vi "XNET BM Iterate Frame Raw to CAN.vi"(5 "index in":i32, 7 "raw frames":u8[](array[numeric]) format="%02x", 11 "error in":errorcluster) -> (4 "output BM Frame":T1={"timestamp"=timestamp(0 s since 1904-01-01), "payload"=[0, 0, 0, 0, 0, 0, 0, 0], "identifier / slot"=0, "Data type"=0, "payload length"=0, "CAN"={"extended?"=FALSE}, "FlexRay"={"cycle count"=0, "startup?"=FALSE, "sync?"=FALSE, "preamble?"=FALSE, "ch A"=FALSE, "ch B"=FALSE, "macrotick"=32}, "echo?"=FALSE} {"FlexRay"."cycle count" max=63 step=1; "payload" format="%x"; "identifier / slot" format="%x"}, 6 "index out":i32, 10 "valid?":bool, 15 "error out":errorcluster)   [LabVIEW 2014, in "CAN Bus Monitor Engine.lvlib"]
doc: "Iterate array of raw frame data to extract a single CAN frame.\n\nIndex in specifies the start of the new CAN frame in the raw data. If no valid frame exists at this index, the boolean \"valid?\" is false.\n\nIndex out specfies the start of the next CAN frame in raw data, or -1 if the end of the raw data was reached.\n\nThis VI is part of the NI-XNET example set."
uses:
  CAN Bus Monitor Engine.lvlib
  Controls/XNET BM Frame.ctl
  <vilib>/xnet/xnet.llb/XNET Frame Type CAN.ctl
  Controls/Set Dyn Vars.ctl
  BM Global Vars.vi
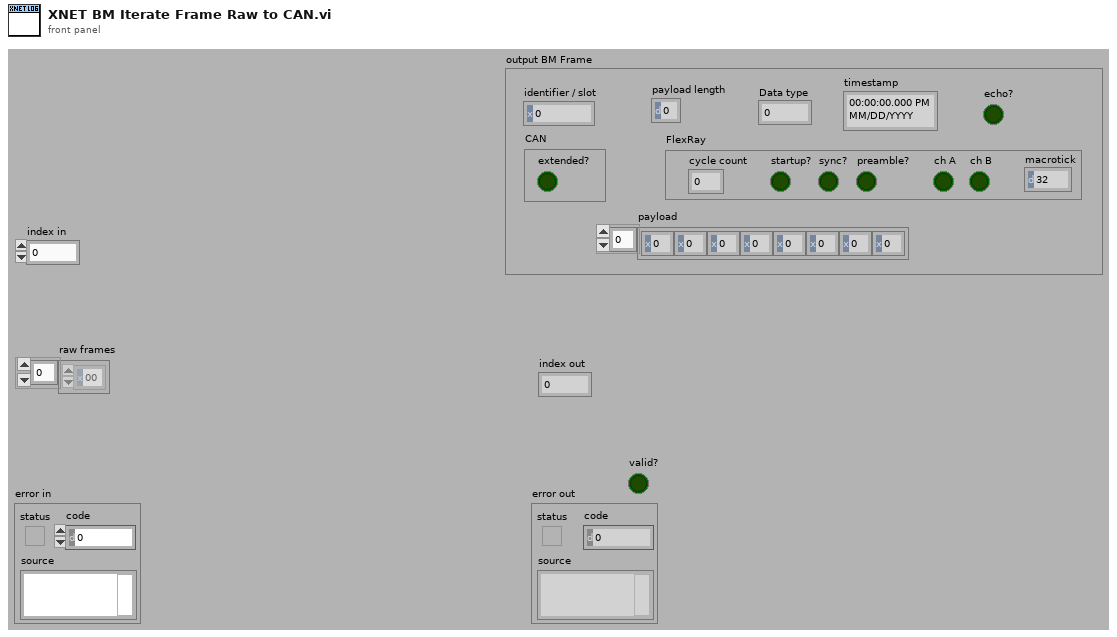
[diagram p1: front panel]
types:
  T1 = typedef "CAN Bus Monitor Engine.lvlib/XNET BM Frame.ctl" = cluster{"timestamp":timestamp, "payload":u8[], "identifier / slot":u32, "Data type":u8, "payload length":u8, "CAN":cluster{"extended?":bool}, "FlexRay":cluster{"cycle count":u8, "startup?":bool, "sync?":bool, "preamble?":bool, "ch A":bool, "ch B":bool, "macrotick":u16}, "echo?":bool}
  T2 = typedef "CAN Bus Monitor Engine.lvlib/Set Dyn Vars.ctl" = enum16{"Std Frames", "Std Frames / Sec", "Ext Frames", "Ext Frames / Sec", "Remote Frames", "Remote Frames / Sec", "Error Frames", "Error Frames / Sec", "BusLoad", "SumFrames", "SumFrames / Sec", "Null Frames", "Null Frames / Sec", "Peak Bus Load", "State", "IncMinFrameTime", "IncMaxFrameTime", "Driver Status", "CAN Comm State", "LIN Comm State", "FlexRay Comm State"}
  T3 = typedef "XNET Frame Type CAN.ctl" = u8
  T4 = enum16{"big-endian, network order", "native, host order", "little-endian"}
  T5 = cluster{"IncMinFrameTime":dbl, "IncMaxFrameTime":dbl, "Min Frame Length":dbl[][], "Max Frame Length":dbl[][], "Std Frames":u32, "Ext Frames":u32, "Error Frames":u32, "Remote Frames":u32, "Std Frames / Sec":u32, "Ext Frames / Sec":u32, "Error Frames / Sec":u32, "Remote Frames / Sec":u32, "Peak Bus Load":dbl, "Bus Load":dbl, "Start Timestamp":dbl, "Null Frames":u32, "Null Frames / Sec":u32}
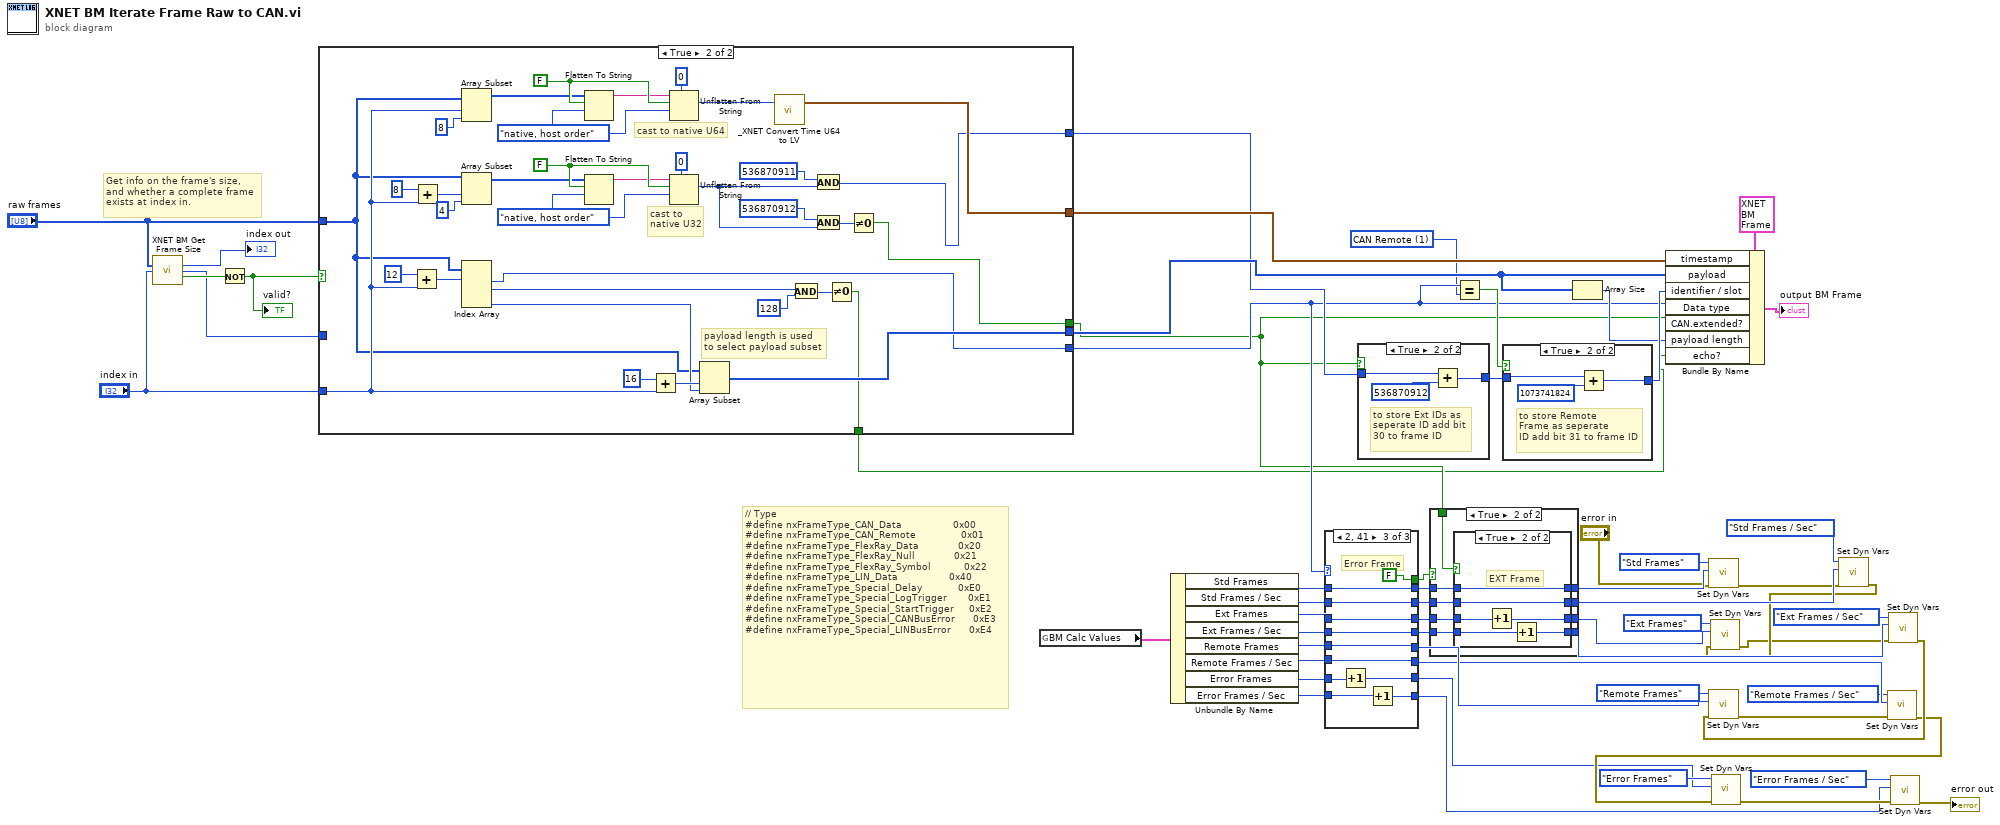
[diagram p0: block diagram]
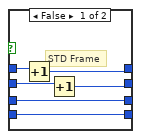
[diagram p3: hidden frame]
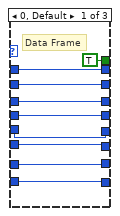
[diagram p6: hidden frame]
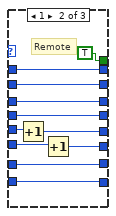
[diagram p7: hidden frame]
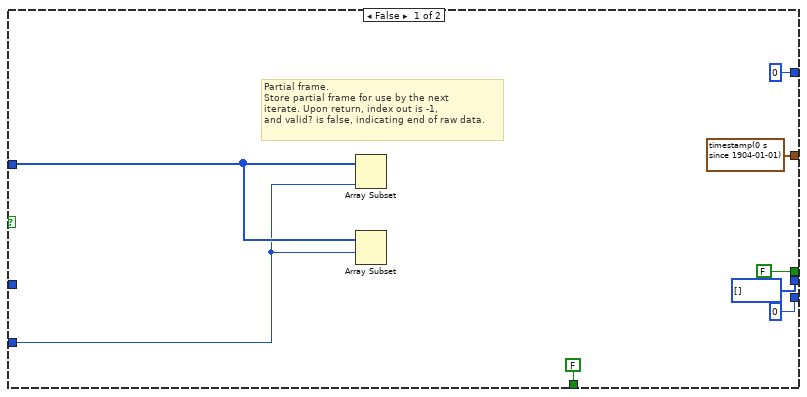
[diagram p8: hidden frame]
diagram:
  w31 = T3 1 items=["CAN Data", "CAN Remote"] ("type")
  # "// Type\n#define nxFrameType_CAN_Data                 0x00\n#define nxFrameType_CAN_Remote               0x01\n#define nxFrameType_FlexRay_Data             0x20\n#define nxFrameType_FlexRay_Null             0x21\n#define nxFrameType_FlexRay_Symbol           0x22\n#define nxFrameType_LIN_Data                 0x40\n#define nxFrameType_Special_Delay            0xE0\n#define nxFrameType_Special_LogTrigger       0xE1\n#define nxFrameType_Special_StartTrigger     0xE2\n#define nxFrameType_Special_CANBusError      0xE3\n#define nxFrameType_Special_LINBusError      0xE4"
  # "Get info on the frame's size,\nand whether a complete frame\nexists at index in."
  n1 = call "XNET BM Get Frame Size.vi"("raw frames"="raw frames", "index"="index in") -> ("next index"=→"index out":i32, "size"=w53:i32, "partial?"=w55:bool)  [unwired: 11 in]
  n2 = Not(x=w55) -> (.not. x?=w54:bool)
  "valid?" <- w54
  n3 = case shown="True" w54 {
    tunnel: "index in" -> [w65 w77]
    tunnel: "raw frames" -> [w66 w76]
    tunnel: w53 -> [_ _]
    tunnel: [timestamp(0 s since 1904-01-01) ("Time LV") w72] -> w37
    tunnel: [u8[] [] w71] -> w36
    tunnel: [u32 0 w70] -> w35
    tunnel: [u8 0 ("Numeric") w69] -> w34
    tunnel: [FALSE w68] -> w33
    tunnel: [FALSE w67] -> w1
    frame False {
      # "Partial frame.\nStore partial frame for use by the next \niterate. Upon return, index out is -1,\nand valid? is false, indicating end of raw data."
      n4 = Array Subset(array=w66, length=w65) -> ()  [unwired: 1 in, 1 out]
      n5 = Array Subset(array=w66, index=w65) -> ()  [unwired: 1 in, 1 out]
    }
    frame True {
      w82 = T4."native, host order" ("byte order (0:big-endian, network order)")
      w88 = T4."native, host order" ("byte order (0:big-endian, network order)")
      w83 = FALSE ("prepend array or string size? (T)")
      w89 = FALSE ("prepend array or string size? (T)")
      # "payload length is used\nto select payload subset"
      # "cast to \nnative U32"
      # "cast to native U64"
      n6 = Add(x=12, y=w77) -> (x+y=w93:i32)
      n7 = Add(x=8, y=w77) -> (x+y=w95:i32)
      n8 = Array Subset(array=w76, index=w77, length=8) -> (w80:u8[])
      n9 = Array Subset(array=w76, index=w95, length=4) -> (w86:u8[])
      n10 = Index Array(array=w76, index #1=w93) -> (element #1=w69:u8, element #2=w73:u8, element #4=w90:u8)  [unwired: 3 in, 1 out]
      n11 = Flatten To String(anything=w80, prepend array or string size? (T)=w83, byte order (0:big-endian, network order)=w82) -> (data string=w81:string)  [unwired: 1 in, 2 out]
      n12 = Flatten To String(anything=w86, prepend array or string size? (T)=w89, byte order (0:big-endian, network order)=w88) -> (data string=w87:string)  [unwired: 1 in, 2 out]
      n13 = Add(x=16, y=w77) -> (x+y=w91:i32)
      n14 = Unflatten From String(type=u64 0 ("length"), binary string=w81, data includes array or string size? (T)=w83, byte order (0:big-endian, network order)=w82) -> (value=w78:u64)  [unwired: 1 in, 2 out]
      n15 = Unflatten From String(type=u32 0 ("length"), binary string=w87, data includes array or string size? (T)=w89, byte order (0:big-endian, network order)=w88) -> (value=w84:u32)  [unwired: 1 in, 2 out]
      n16 = Array Subset(array=w76, index=w91, length=w90) -> (w71:u8[])
      n17 = call <vilib>:"_XNET Convert Time U64 to LV.vi"("Time U64"=w78) -> ("Time LV"=w72:timestamp)  [unwired: 2 in]
      n18 = And(x=w73, y=u8 128) -> (x .and. y?=w75:u8)
      n19 = And(x=u32 536870911, y=w84) -> (x .and. y?=w70:u32)
      n20 = And(x=u32 536870912, y=w84) -> (x .and. y?=w99:u32)
      n21 = Not Equal To 0?(x=w75) -> (x != 0?=w67:bool)
      n22 = Not Equal To 0?(x=w99) -> (x != 0?=w68:bool)
    }
  }
  n23 = global read "BM Global Vars.vi" "BM Calc Values"() -> (w30:T5)
  n24 = Unbundle By Name(w30) -> ("Std Frames"=w52:u32, "Std Frames / Sec"=w51:u32, "Ext Frames"=w50:u32, "Ext Frames / Sec"=w49:u32, "Remote Frames"=w48:u32, "Remote Frames / Sec"=w47:u32, "Error Frames"=w11:u32, "Error Frames / Sec"=w10:u32)
  n25 = case shown="2, 41" w34 {
    tunnel: w50 -> [w106 w119 w130]
    tunnel: w49 -> [w105 w118 w129]
    tunnel: w52 -> [w108 w121 w132]
    tunnel: [w108 w121 w132] -> w42
    tunnel: [w107 w120 w131] -> w41
    tunnel: w51 -> [w107 w120 w131]
    tunnel: [w106 w119 w130] -> w40
    tunnel: [w105 w118 w129] -> w39
    tunnel: w48 -> [w109 w117 w128]
    tunnel: w47 -> [w110 w116 w127]
    tunnel: [w109 w115 w128] -> w26
    tunnel: [w110 w114 w127] -> w25
    tunnel: w11 -> [w104 w113 w126]
    tunnel: w10 -> [w103 w112 w125]
    tunnel: [w104 w113 w124] -> w4
    tunnel: [w103 w112 w123] -> w3
    tunnel: [TRUE TRUE FALSE] -> w2
    frame 0, Default {
      # "Data Frame"
    }
    frame 1 {
      # "Remote"
      n26 = Increment(x=w117) -> (x+1=w115:u32)
      n27 = Increment(x=w116) -> (x+1=w114:u32)
    }
    frame 2, 65 {
      # "Error Frame"
      n28 = Increment(x=w126) -> (x+1=w124:u32)
      n29 = Increment(x=w125) -> (x+1=w123:u32)
    }
  }
  n30 = case shown="True" w33 {
    tunnel: w35 -> [w133 w135]
    tunnel: [w133 w136] -> w46
    frame False {
    }
    frame True {
      # "to store Ext IDs as\nseperate ID add bit \n30 to frame ID"
      n31 = Add(x=w135, y=u32 536870912) -> (x+y=w136:u32)
    }
  }
  n32 = case shown="True" w2 {
    tunnel: w42 -> [w140 w149]
    tunnel: w41 -> [w139 w148]
    tunnel: w40 -> [w138 w147]
    tunnel: w39 -> [w137 w146]
    tunnel: w33 -> [_ w145]
    tunnel: [w140 w144] -> w29
    tunnel: [w139 w143] -> w28
    tunnel: [w138 w142] -> w27
    tunnel: [w137 w141] -> w24
    frame False {
    }
    frame True {
      n33 = case shown="True" w145 {
        tunnel: w146 -> [w155 w161]
        tunnel: [w154 w160] -> w142
        tunnel: [w155 w159] -> w141
        tunnel: w147 -> [w154 w158]
        tunnel: w149 -> [w153 w157]
        tunnel: [w152 w157] -> w144
        tunnel: [w150 w156] -> w143
        tunnel: w148 -> [w151 w156]
        frame False {
          # "STD Frame"
          n34 = Increment(x=w153) -> (x+1=w152:u32)
          n35 = Increment(x=w151) -> (x+1=w150:u32)
        }
        frame True {
          # "EXT Frame"
          n36 = Increment(x=w158) -> (x+1=w160:u32)
          n37 = Increment(x=w161) -> (x+1=w159:u32)
        }
      }
    }
  }
  n38 = Equal?(x=w34, y=w31) -> (x = y?=w44:bool)
  n39 = case shown="True" w44 {
    tunnel: w46 -> [w162 w164]
    tunnel: [w162 w165] -> w45
    frame False {
    }
    frame True {
      # "to store Remote \nFrame as seperate \nID add bit 31 to frame ID"
      n40 = Add(x=w164, y=u32 1073741824) -> (x+y=w165:u32)
    }
  }
  n41 = Array Size(array=w36) -> (size(s)=w43:i32)
  n42 = Bundle By Name(cluster=T1 {"timestamp"=timestamp(0 s since 1904-01-01), "payload"=[0, 0, 0, 0, 0, 0, 0, 0], "identifier / slot"=0, "Data type"=0, "payload length"=0, "CAN"={"extended?"=FALSE}, "FlexRay"={"cycle count"=0, "startup?"=FALSE, "sync?"=FALSE, "preamble?"=FALSE, "ch A"=FALSE, "ch B"=FALSE, "macrotick"=0}, "echo?"=FALSE} ("CAN frame"), "timestamp"=w37, "payload"=w36, "identifier / slot"=w45, "Data type"=w34, "CAN.extended?"=w33, "payload length"=w43, "echo?"=w1) -> (→"output BM Frame":T1)
  n43 = call "Set Dyn Vars.vi"("error in"="error in", "Data"=w29, "Set Values"=Set_Dyn_Vars."Std Frames") -> ("error out"=w16:errorcluster)  [unwired: 8 in]
  n44 = call "Set Dyn Vars.vi"("error in"=w16, "Data"=w28, "Set Values"=Set_Dyn_Vars."Std Frames / Sec") -> ("error out"=w15:errorcluster)  [unwired: 8 in]
  n45 = call "Set Dyn Vars.vi"("error in"=w15, "Data"=w27, "Set Values"=Set_Dyn_Vars."Ext Frames") -> ("error out"=w14:errorcluster)  [unwired: 8 in]
  n46 = call "Set Dyn Vars.vi"("error in"=w14, "Data"=w24, "Set Values"=Set_Dyn_Vars."Ext Frames / Sec") -> ("error out"=w13:errorcluster)  [unwired: 8 in]
  n47 = call "Set Dyn Vars.vi"("error in"=w13, "Data"=w26, "Set Values"=Set_Dyn_Vars."Remote Frames") -> ("error out"=w12:errorcluster)  [unwired: 8 in]
  n48 = call "Set Dyn Vars.vi"("error in"=w12, "Data"=w25, "Set Values"=Set_Dyn_Vars."Remote Frames / Sec") -> ("error out"=w5:errorcluster)  [unwired: 8 in]
  n49 = call "Set Dyn Vars.vi"("error in"=w5, "Data"=w4, "Set Values"=Set_Dyn_Vars."Error Frames") -> ("error out"=w9:errorcluster)  [unwired: 8 in]
  n50 = call "Set Dyn Vars.vi"("error in"=w9, "Data"=w3, "Set Values"=Set_Dyn_Vars."Error Frames / Sec") -> ("error out"=→"error out":errorcluster)  [unwired: 8 in]
